vi "Meas Panel Multi Freq Sweep.vi"(8 "error in (no error)":errorcluster) -> (0 "error out":errorcluster, 3 "freq lst out":dbl[](array[numeric]) caption="Frequency list [Hz]" format="%#_6p")   [LabVIEW 2013]
doc: "Select multi-frequency list for multi-frequency sweeps."
panel:
  in  "btn ok":bool
  in  "btn flst clr":bool
  in  "freq lst":dbl[](array[numeric]) caption="Frequency list [Hz]" format="%#_6p"
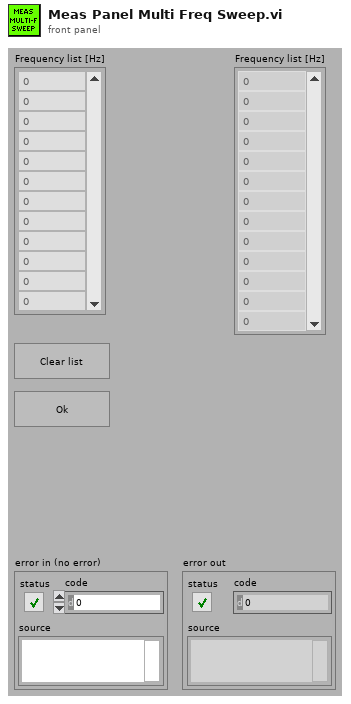
[diagram p1: front panel]
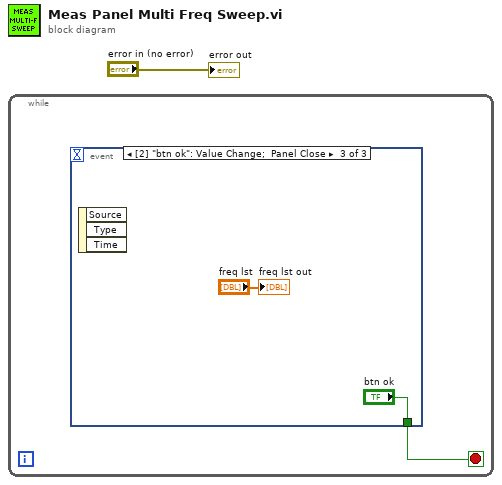
[diagram p0: block diagram]
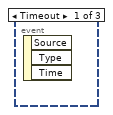
[diagram p2: hidden frame]
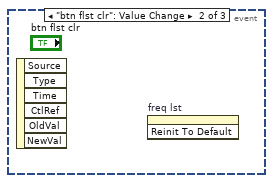
[diagram p3: hidden frame]
diagram:
  n1 = while {
    stop <- w2 stop-if-true
    n2 = event shown="[2] \"btn ok\": Value Change;  Panel Close" {
      selector: _ -> [_ _ _]
      dyn-events: _ -> [_ _ _]
      timeout: _ -> [_ _ _]
      tunnel: [_ _ "btn ok"] -> w2
      event Timeout {
        n3 = event-data() -> ()  [unwired: 1 in, 3 out]
      }
      event "btn flst clr": Value Change {
        n4 = event-data() -> ()  [unwired: 1 in, 6 out]
        n5 = invoke on="freq lst" class="Arr (strict)" method="Reinit To Default"() -> ()  [unwired: 3 in, 3 out]
      }
      event "btn ok": Value Change; Panel Close {
        n6 = event-data() -> ()  [unwired: 1 in, 3 out]
        "freq lst out" <- "freq lst"
      }
    }
  }
  "error out" <- "error in (no error)"
